vi "GUI_FrogHPD.vi"() -> ()   [LabVIEW 2013]
uses:
  GUI_Template/GUI_master/tcp_new_data_event.ctl
  GUI_Template/GUI_master/tcp new data cluster.ctl
  <vilib>/vision/Image Controls.llb/IMAQ Image.ctl
panel:
  out "SpatialImage::1":T1(plugin-control) caption="Spatial Image"
  in  "triggermode::1":T2(ring)
  out "retrievedFrogTrace::1":T1(plugin-control) caption="Retrieved Frog Trace"
  out "temporalFWHM::1":dbl caption="Pulse Width" min=0.0 max=50000.0
  out "frogTrace::1":T1(plugin-control) caption="FROG Trace"
  in  "exposure::1":dbl=0.001 caption="Exposure" min=0.0453 max=10000.0 format="%_4p"
  in  "insert tag":bool=TRUE
  in  "stop":bool
  in  "GUIdevice 1":string="FrogHPD"
  out "tcp data event":T3
  out "error IO 2":errorcluster
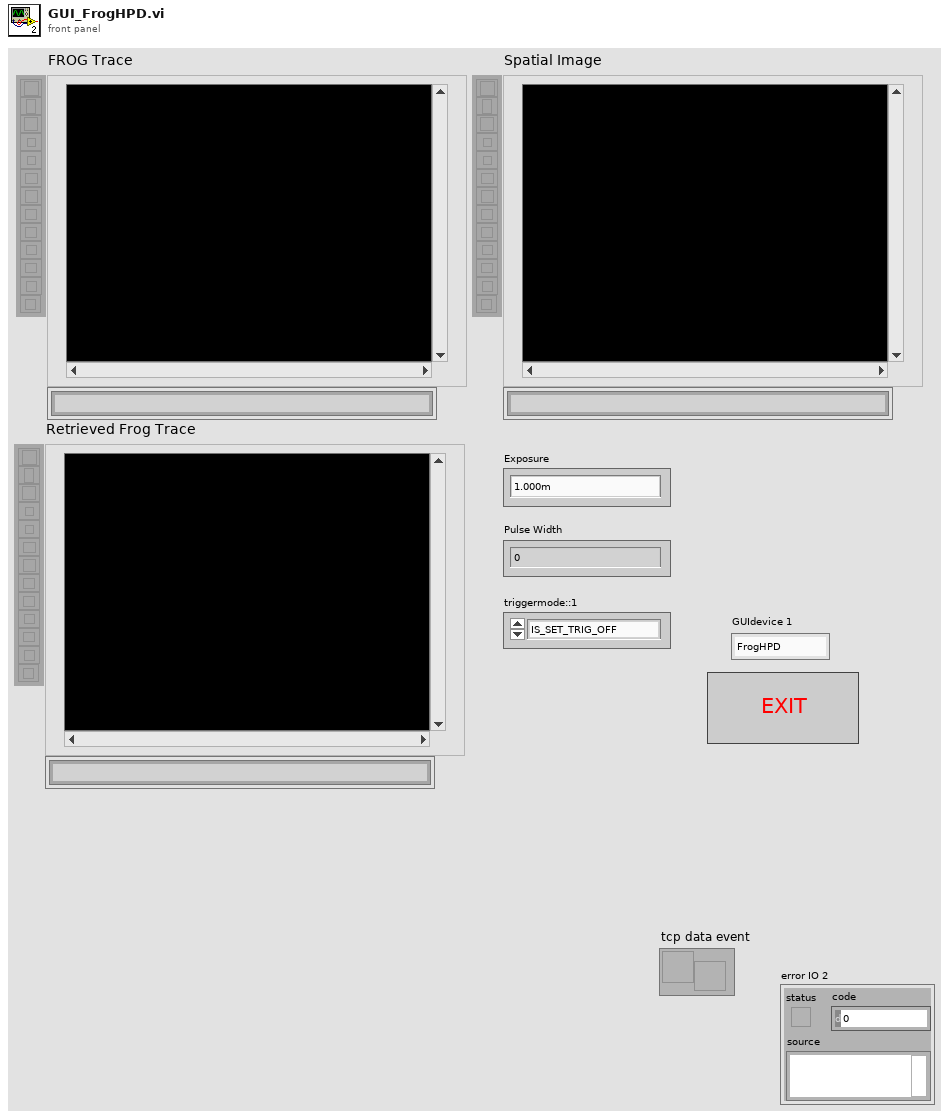
[diagram p1: front panel]
types:
  T1 = typedef "IMAQ Image.ctl" = refnum<image>
  T2 = enum16{"IS_SET_TRIG_OFF", "IS_SET_TRIG_HI_LO", "IS_SET_TRIG_LO_HI", "IS_SET_TRIG_SOFTWARE", "IS_GET_EXTERNAL_TRIGGER", "IS_GET_TRIGGER_STATUS"}
  T3 = typedef "tcp_new_data_event.ctl" = refnum<user-event>
  T4 = typedef "tcp new data cluster.ctl" = cluster{"EventEnum":enum16{"new data", "connection status update"}, "Device name":string}
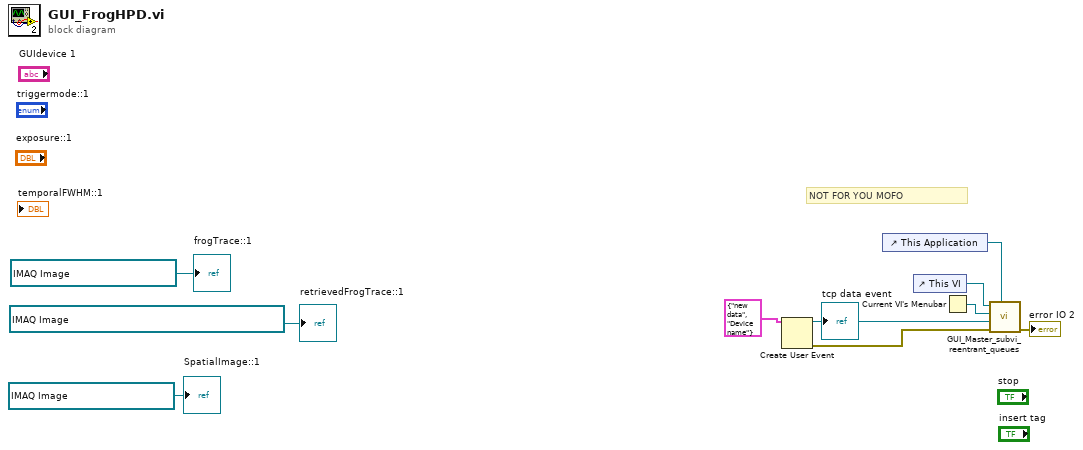
[diagram p0: block diagram]
diagram:
  # "NOT FOR YOU MOFO"
  n1 = Create User Event(user event datatype=T4 {"EventEnum"=enum."new data", "Device name"="Device name"} ("New Event")) -> (user event=w5:refnum<user-event>, error out=w6:errorcluster)  [unwired: 1 in]
  "tcp data event" <- w5
  n2 = control-ref of="This Application"() -> (w1:refnum<vi>)
  n3 = control-ref of="This VI"() -> (w9:refnum<vi>)
  n4 = Current VI's Menubar() -> (w8:refnum<k9>)
  n5 = call "GUI_Master_subvi_reentrant_queues.vi"("This Application"=w1, "error in (no error)"=w6, "tcp data event"=w5, "Caller menu reference"=w8, "Caller VI ref"=w9) -> ("error out"=→"error IO 2":errorcluster)  [unwired: 6 in]
  "frogTrace::1" <- T1 refnum ("New Image")
  "retrievedFrogTrace::1" <- T1 refnum ("New Image")
  "SpatialImage::1" <- T1 refnum ("New Image")
